vi "create_menu.vi"(8 "error in (no error)":errorcluster, 9 "lookup string":string, 10 "Menus":string[][](array[string])=[["item0", "<submenu0>"], ["item1", "submenuitem0"], ["<submenu0>", ""]], 11 "BalloonNotifier in":refnum<class "BalloonNotifier.lvclass">) -> (0 "error out":errorcluster, 2 "MenuItem references":refnum<k24>[](array[refnum]), 3 "BalloonNotifier out":refnum<class "BalloonNotifier.lvclass">)   [LabVIEW 2017, in "BalloonNotifier.lvclass"]
uses:
  BalloonNotifier.lvclass
  System.Windows.Forms
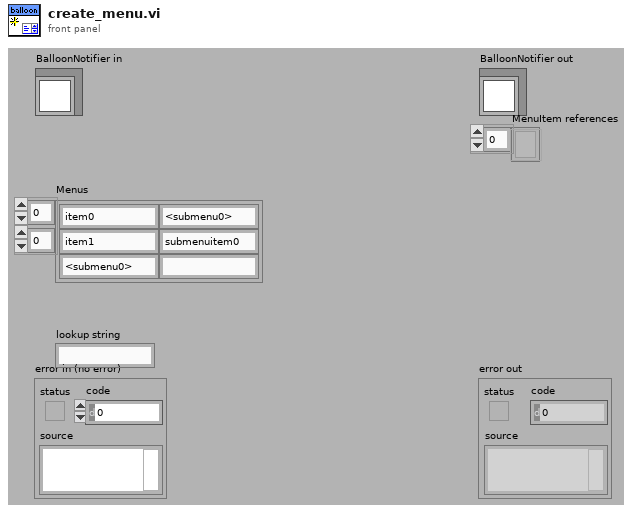
[diagram p1: front panel]
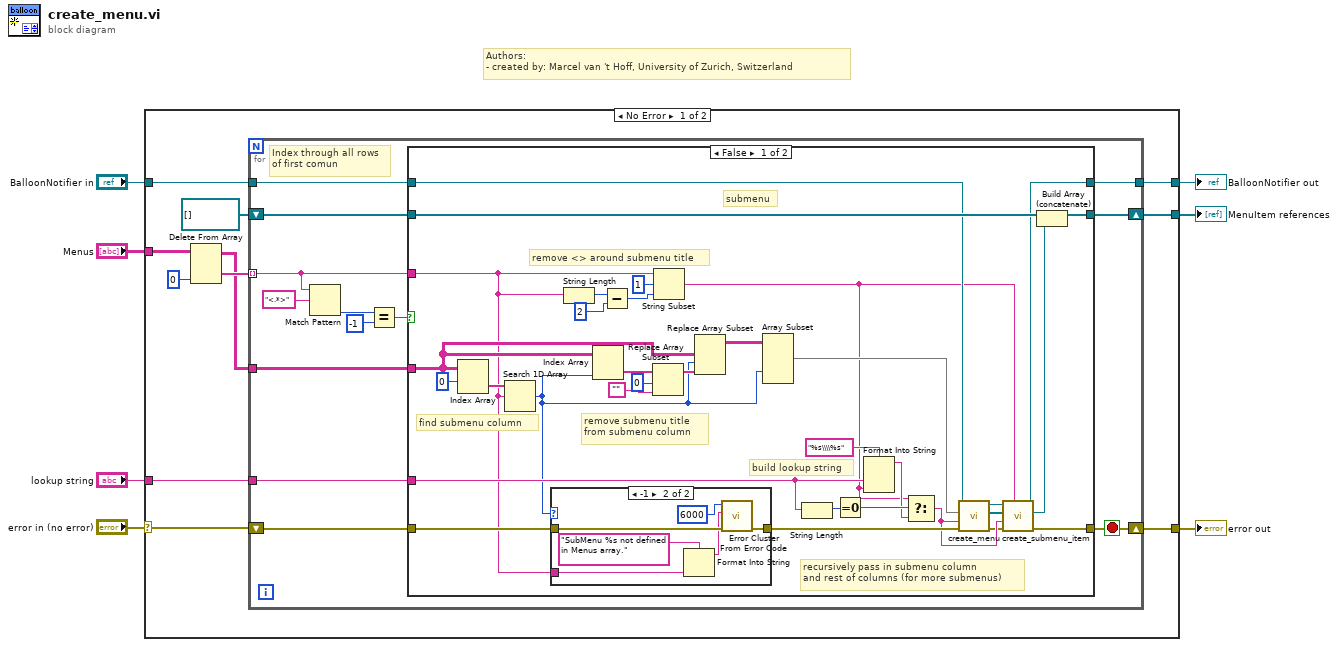
[diagram p0: block diagram]
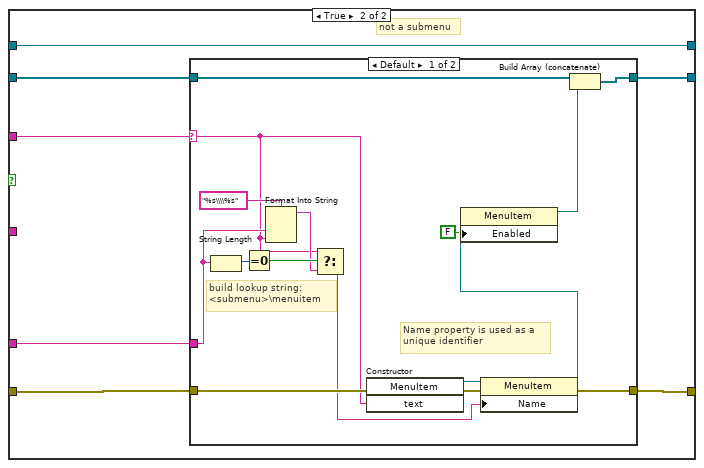
[diagram p3: hidden frame]
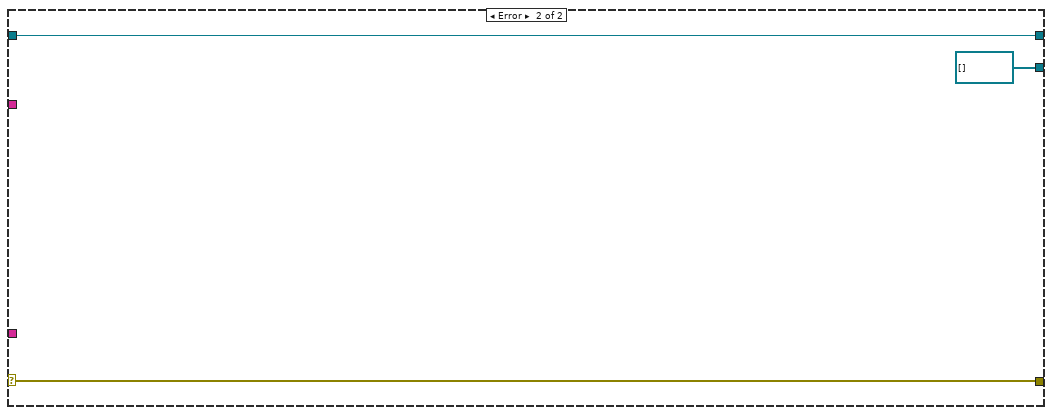
[diagram p5: hidden frame]
diagram:
  # "Authors: \n- created by: Marcel van 't Hoff, University of Zurich, Switzerland"
  n1 = case shown="No Error" "error in (no error)" {
    selector: "error in (no error)" -> [w14 w99]
    tunnel: [w18 refnum<k24>[] []] -> w1
    tunnel: "Menus" -> [w13 _]
    tunnel: [w16 w99] -> w7
    tunnel: "lookup string" -> [w15 _]
    tunnel: "BalloonNotifier in" -> [w9 w97]
    tunnel: [w8 w97] -> w2
    frame No Error {
      n2 = Delete From Array(array=w13, index (col)=0 ("disabled index (col)")) -> (deleted portion=w11:string[], array with subset deleted=w10:string[][])  [unwired: 2 in]
      n3 = for {
        tunnel: w11 -> [w27] mode=indexing
        shift-right: [w26] -> w18
        shift-left: refnum<k24>[] [] -> [w25]
        tunnel: w10 -> [w24]
        tunnel: w15 -> [w22]
        shift-right: [w21] -> w16
        shift-left: w14 -> [w23]
        tunnel: w9 -> [w20]
        tunnel: [w19] -> w8
        stop <- w21 stop-if-true
        # "Index through all rows\nof first comun"
        n4 = Match Pattern(string=w27, regular expression="<.*>") -> (offset past match=w30:i32)  [unwired: 1 in, 3 out]
        n5 = Equal?(x=w30, y=-1) -> (x = y?=w28:bool)
        n6 = case shown="False" w28 {
          tunnel: w27 -> [w43 w74]
          tunnel: [w58 w78] -> w26
          tunnel: w25 -> [w57 w77]
          tunnel: w24 -> [w55 _]
          tunnel: w23 -> [w44 w76]
          tunnel: [w34 w75] -> w21
          tunnel: w22 -> [w49 w73]
          tunnel: w20 -> [w42 w72]
          tunnel: [w32 w72] -> w19
          frame False {
            # "build lookup string"
            # "recursively pass in submenu column\nand rest of columns (for more submenus)"
            # "remove submenu title\nfrom submenu column"
            # "find submenu column"
            # "remove <> around submenu title"
            # "submenu"
            n7 = Index Array(array=w55, index (row)=0) -> (element=w59:string[])  [unwired: 1 in]
            n8 = Search 1D Array(1D array=w59, element=w43) -> (index of element=w45:i32)  [unwired: 1 in]
            n9 = case shown="-1" w45 {
              tunnel: w44 -> [w65 w71]
              tunnel: [w65 w70] -> w40
              tunnel: w43 -> [_ w68]
              frame 0, Default {
              }
              frame -1 {
                n10 = Format Into String(format string="SubMenu %s not defined in Menus array." ("error message (\"\")"), w68) -> (resulting string=w67:string)  [unwired: 2 in, 1 out]
                n11 = call <vilib>:"Error Cluster From Error Code.vi"("error in (no error)"=w71, "error message (\"\")"=w67, "error code (0)"=6000) -> ("error out"=w70:errorcluster)  [unwired: 6 in]
              }
            }
            n12 = String Length(string=w43) -> (length=w62:i32)
            n13 = Index Array(array=w55, index (col)=w45) -> (element=w56:string[])  [unwired: 1 in]
            n14 = Subtract(x=w62, y=2) -> (x-y=w60:i32)
            n15 = Replace Array Subset(array=w56, new element="", index=0) -> (w54:string[])
            n16 = String Subset(string=w43, offset (0)=1, length (rest)=w60) -> (substring=w38:string)
            n17 = Replace Array Subset(array=w55, new element=w54, index (col)=w45) -> (w53:string[][])  [unwired: 1 in]
            n18 = Array Subset(array=w53, index (col)=w45) -> (w41:string[][])  [unwired: 3 in]
            n19 = String Length(string=w49) -> (length=w48:i32)
            n20 = Equal To 0?(x=w48) -> (x = 0?=w47:bool)
            n21 = Format Into String(format string="%s\\\\%s", w49, w38) -> (resulting string=w46:string)  [unwired: 2 in, 1 out]
            n22 = Select(t=w38, s=w47, f=w46) -> (s? t:f=w37:string)
            n23 = call-dynamic "create_menu.vi"("error in (no error)"=w40, "lookup string"=w37, "Menus"=w41, "BalloonNotifier in"=w42) -> ("error out"=w35:errorcluster, "MenuItem references"=w36:refnum<k24>[], "BalloonNotifier out"=w39:refnum<class "BalloonNotifier.lvclass">)  [unwired: 5 in]
            n24 = call-dynamic "create_submenu_item.vi"("SubMenu Title"=w38, "error in (no error)"=w35, "lookup string"=w37, "MenuItem references"=w36, "BalloonNotifier in"=w39) -> ("error out"=w34:errorcluster, "SubMenuItem reference"=w33:refnum<k24>, "BalloonNotifier out"=w32:refnum<class "BalloonNotifier.lvclass">)  [unwired: 4 in]
            n25 = Build Array (concatenate)(w57, w33) -> (w58:refnum<k24>[])
          }
          frame True {
            # "not a submenu"
            n26 = case shown="Default" w74 {
              selector: w74 -> [w83 _]
              tunnel: [w94 w96] -> w78
              tunnel: w77 -> [w93 w96]
              tunnel: w76 -> [w92 w95]
              tunnel: [w89 w95] -> w75
              tunnel: w73 -> [w84 _]
              frame Default {
                # "Name property is used as a \nunique identifier"
                # "build lookup string:\n<submenu>\\menuitem"
                n27 = String Length(string=w84) -> (length=w87:i32)
                n28 = Equal To 0?(x=w87) -> (x = 0?=w86:bool)
                n29 = Format Into String(format string="%s\\\\%s", w84, w83) -> (resulting string=w85:string)  [unwired: 2 in, 1 out]
                n30 = Select(t=w83, s=w86, f=w85) -> (s? t:f=w82:string)
                n31 = constructor class="MenuItem"(error in=w92, "text"=w83) -> (reference out=w91:refnum<k24>, error out=w90:errorcluster)  [unwired: 2 in, 2 out]
                n32 = property class="MenuItem"(reference=w91, error in=w90, "Name"=w82) -> (reference out=w80:refnum<k24>, error out=w89:errorcluster)
                n33 = property class="MenuItem"(reference=w80, "Enabled"=FALSE) -> (reference out=w81:refnum<k24>)  [unwired: 1 in, 1 out]
                n34 = Build Array (concatenate)(w93, w81) -> (w94:refnum<k24>[])
              }
              frame "" {
                # "skip empty strings\ncreated for 2D array"
              }
            }
          }
        }
      }
    }
    frame Error {
    }
  }
  "error out" <- w7
  "BalloonNotifier out" <- w2
  "MenuItem references" <- w1
